vi "GDSAPI_GetMethodOptions.vi"(8 "error in (no error)":errorcluster, 10 "OriginalClassPath(*.lvclass)":path) -> (0 "error out":errorcluster, 1 "PropertyMethodTemplates":string[](array[string]), 2 "OverrideMethodTemplates":string[](array[string]), 3 "NormalMethodTemplates":string[](array[string]), 4 "AllDynamicMethodsToOverride":path[](array[path]), 6 "Properties":string[](array[string]))   [LabVIEW 2020]
doc: "This VI could be used to view the possible options that are available when creating methods in a class, using the API VI \"CreateMethods.vi\","
uses:
  <resource>/Framework/Providers/Open_GDS/ClassProviders/Provider_LvNativeClass/ClassWriterNative_class/ClassWriterNative.lvclass
panel:
  in  "Tree":string(tree)
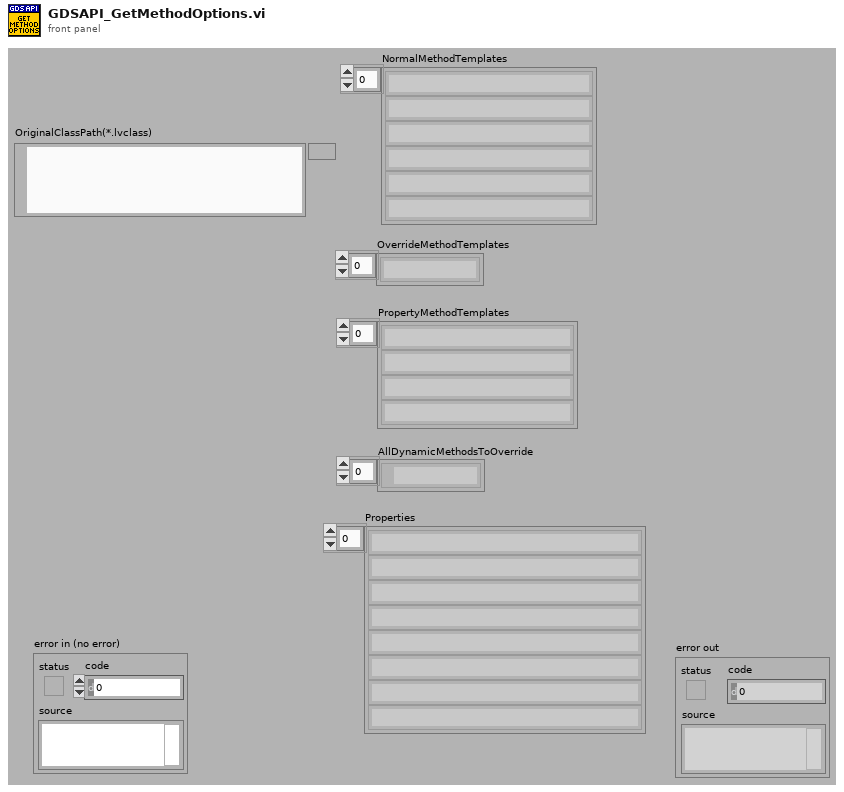
[diagram p1: front panel]
types:
  T1 = typedef "GDSLvCLass_ClassSettingsType.ctl" = cluster{"ClassProviderName":string, "ClassTemplateUsed":string, "ClassTemplateVersion":string, "ClassDescription":string, "PlugIns":T2[], "ConnectorPanePattern":string}
  T2 = typedef "GDSLvClass_PlugIn.ctl" = cluster{"Type":T3, "ID":string, "Version":string, "Path":path, "Name":string, "Data":variant}
  T3 = typedef "GDSLvClass_PlugInTypes.ctl" = enum16{"DesignPattern", "MethodTypes"}
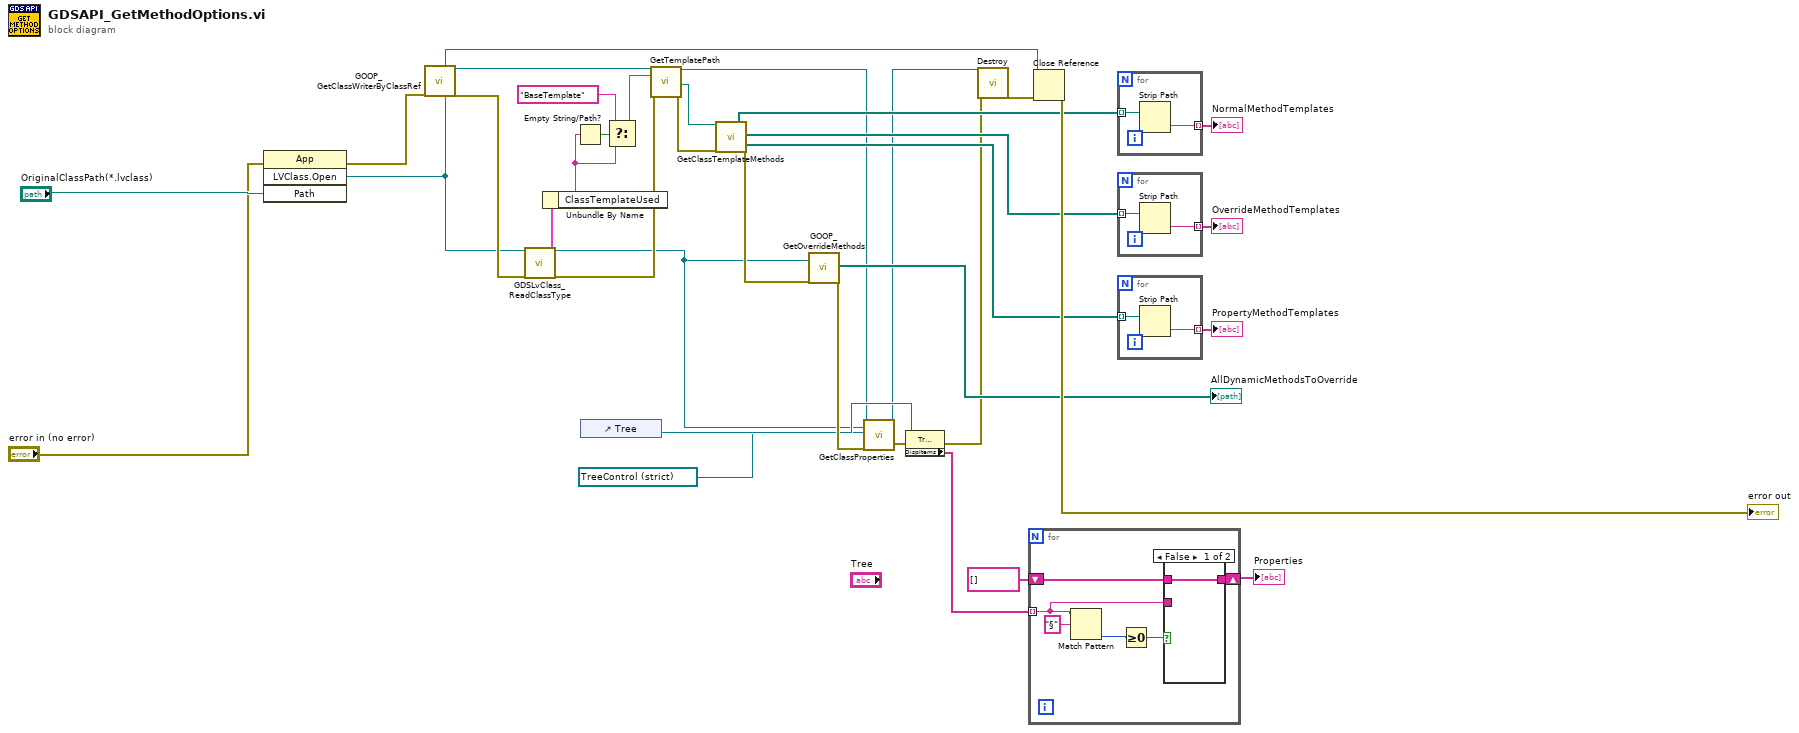
[diagram p0: block diagram]
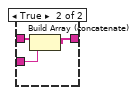
[diagram p2: hidden frame]
diagram:
  n1 = invoke class="App" method="LVClass.Open"(error in="error in (no error)", "Path"="OriginalClassPath(*.lvclass)") -> (error out=w31:errorcluster, "LVClass.Open"=w29:refnum<vi>)  [unwired: 2 in, 2 out]
  n2 = call <resource>:"GOOP_GetClassWriterByClassRef.vi"("LVClassLibrary Refnum"=w29, "error in (no error)"=w31) -> ("ClassWriterNative.lvclass"=w28:refnum<class "ClassWriterNative.lvclass">, "error out"=w30:errorcluster)  [unwired: 16 in]
  n3 = call <resource>:"GDSLvClass_ReadClassType.vi"("Class Refnum In"=w29, "error in (no error)"=w30) -> ("Class Refnum Out"=w5:refnum<vi>, "ClassSettings"=w25:T1, "error out"=w21:errorcluster)  [unwired: 15 in]
  n4 = Unbundle By Name(w25) -> ("ClassTemplateUsed"=w24:string)
  n5 = Empty String/Path?(string/path=w24) -> (empty?=w27:bool)
  n6 = control-ref of="Tree"() -> (w9:refnum<vi>)
  n7 = Select(t="BaseTemplate", s=w27, f=w24) -> (s? t:f=w23:string)
  n8 = call-dynamic "GetTemplatePath.vi"("reference in"=w28, "ClassTemplateSubDirectory"=w23, "error in (no error)"=w21) -> ("reference out"=w7:refnum<class "ClassWriterNative.lvclass">, "MethodTemplatePathOut"=w22:path, "error out"=w20:errorcluster)  [unwired: 12 in, 2 out]
  n9 = call <resource>:"GetClassTemplateMethods.vi"("MethodTemplatePath"=w22, "error in"=w20) -> ("NormalMethodPaths"=w19:path[], "OverrideMethodPaths"=w15:path[], "PropertyMethodPaths"=w14:path[], "error out"=w13:errorcluster)  [unwired: 7 in, 7 out]
  n10 = call <resource>:"GOOP_GetOverrideMethods.vi"("LvClassItem"=w5, "error in (no error)"=w13) -> ("DynamicMehods(Paths)"=→"AllDynamicMethodsToOverride":path[], "error out"=w11:errorcluster)  [unwired: 12 in, 4 out]
  n11 = call-dynamic "GetClassProperties.vi"("reference in"=w7, "LvClassItem"=w5, "TreeControl"=refnum<vi> refnum, "error in (no error)"=w11) -> ("reference out"=w6:refnum<class "ClassWriterNative.lvclass">, "error out"=w10:errorcluster)  [unwired: 14 in]
  n12 = property class="Tree (strict)"(reference=w9, error in=w10) -> (error out=w8:errorcluster, "DispItems"=w4:string[])  [unwired: 1 out]
  n13 = call-dynamic "Destroy.vi"("ClassWriterNative"=w6, "error in (no error)"=w8) -> ("error out"=w32:errorcluster)  [unwired: 17 in]
  n14 = for {
    tunnel: w4 -> [w38] mode=indexing
    shift-right: [w36] -> w2
    shift-left: string[] [] -> [w37]
    n15 = Match Pattern(string=w38, regular expression="§") -> (offset past match=w40:i32)  [unwired: 1 in, 3 out]
    n16 = Greater Or Equal To 0?(x=w40) -> (x >= 0?=w39:bool)
    n17 = case shown="False" w39 {
      tunnel: w38 -> [_ w45]
      tunnel: w37 -> [w42 w44]
      tunnel: [w42 w43] -> w36
      frame False {
      }
      frame True {
        n18 = Build Array (concatenate)(w44, w45) -> (w43:string[])
      }
    }
  }
  "Properties" <- w2
  n19 = Close Reference(reference=w29, error in (no error)=w32) -> (error out=→"error out":errorcluster)
  n20 = for {
    tunnel: w19 -> [w47] mode=indexing
    tunnel: [w46] -> w18 mode=indexing
    n21 = Strip Path(path=w47) -> (name=w46:string)  [unwired: 1 out]
  }
  "NormalMethodTemplates" <- w18
  n22 = for {
    tunnel: w15 -> [w49] mode=indexing
    tunnel: [w48] -> w17 mode=indexing
    n23 = Strip Path(path=w49) -> (name=w48:string)  [unwired: 1 out]
  }
  "OverrideMethodTemplates" <- w17
  n24 = for {
    tunnel: w14 -> [w51] mode=indexing
    tunnel: [w50] -> w16 mode=indexing
    n25 = Strip Path(path=w51) -> (name=w50:string)  [unwired: 1 out]
  }
  "PropertyMethodTemplates" <- w16
